vi "Process Pulse.vi"(8 "error in (no error)":errorcluster, 10 "Input":T2={"From"="broadcaster", "To"="broadcaster", "Pulse"=FALSE}, 11 "Flipflop in":refnum<class "Flipflop.lvclass">) -> (0 "error out":errorcluster, 2 "Outputs":T1(array[cluster]), 3 "Flipflop out":refnum<class "Flipflop.lvclass">)   [LabVIEW 2021, in "Flipflop.lvclass"]
uses:
  Flipflop.lvclass
  Flipflop.lvclass/Flipflop.ctl
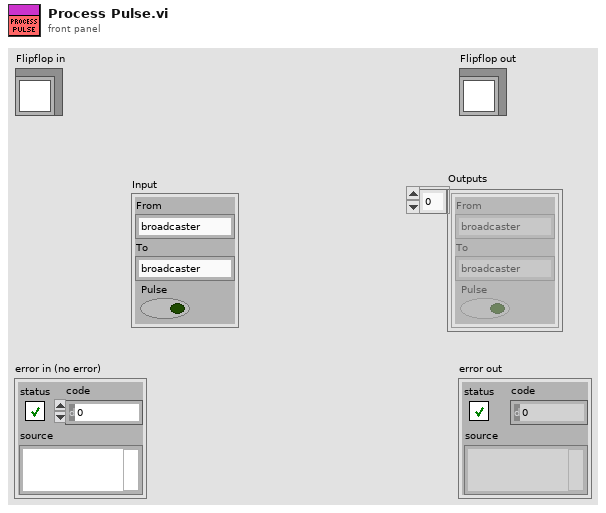
[diagram p1: front panel]
types:
  T1 = cluster{"From":string, "To":string, "Pulse":bool}[]
  T2 = cluster{"From":string, "To":string, "Pulse":bool}
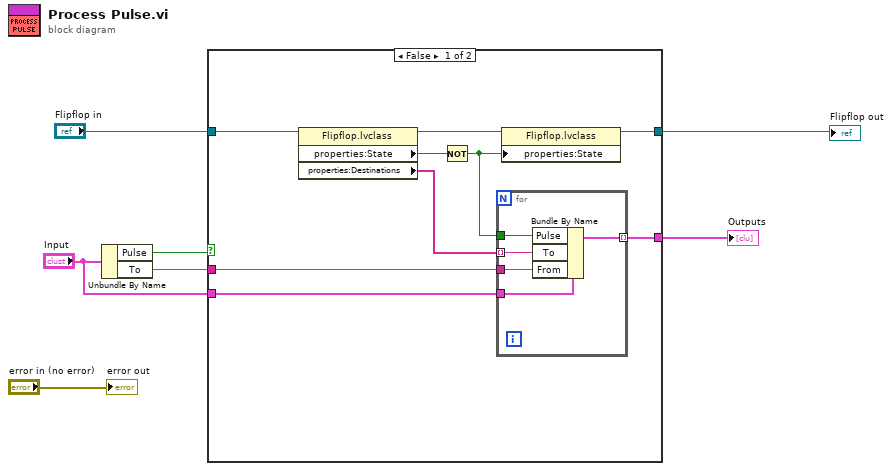
[diagram p0: block diagram]
diagram:
  n1 = Unbundle By Name("Input") -> ("Pulse"=w6:bool, "To"=w2:string)
  n2 = case shown="False" w6 {
    tunnel: "Flipflop in" -> [w15 w22]
    tunnel: [w16 w22] -> w5
    tunnel: [w11 _] -> w4
    tunnel: w2 -> [w8 _]
    tunnel: "Input" -> [w9 _]
    frame False {
      n3 = property class="Flipflop.lvclass"(reference=w15) -> (reference out=w14:refnum<class "Flipflop.lvclass">, "properties:State"=w13:bool, "properties:Destinations"=w10:string[])  [unwired: 1 in, 1 out]
      n4 = Not(x=w13) -> (.not. x?=w12:bool)
      n5 = for {
        tunnel: w12 -> [w21]
        tunnel: [w20] -> w11 mode=indexing
        tunnel: w10 -> [w19] mode=indexing
        tunnel: w9 -> [w18]
        tunnel: w8 -> [w17]
        n6 = Bundle By Name(cluster=w18, "Pulse"=w21, "To"=w19, "From"=w17) -> (w20:T2)
      }
      n7 = property class="Flipflop.lvclass"(reference=w14, "properties:State"=w12) -> (reference out=w16:refnum<class "Flipflop.lvclass">)  [unwired: 1 in, 1 out]
    }
    frame True {
    }
  }
  "Flipflop out" <- w5
  "Outputs" <- w4
  "error out" <- "error in (no error)"
